vi "Launcher (Top Level).vi"(8 "Error In":errorcluster) -> (0 "Error Out":errorcluster)   [LabVIEW 2015]
doc: "This VI is used to launch all modules to run in parallel. Each module has APIs to do its own operation \nand send and receive data from other modules."
uses:
  User Events/Controls/User Events States.ctl
  Modules/Config Database/Config DB.lvlib
  Modules/Vehicle Position Interface/Vehicle Position Interface.lvlib
  Modules/Wash Display Console/Wash Display Console.lvlib
  Modules/Entry Console/Entry Console.lvlib
  Modules/Controller/Controller.lvlib
  Modules/Error Handler/Error Handler.lvlib
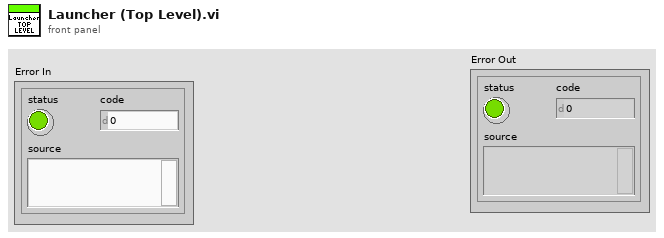
[diagram p1: front panel]
types:
  T1 = typedef "User Events States.ctl" = enum16{"Get", "Create", "Destroy"}
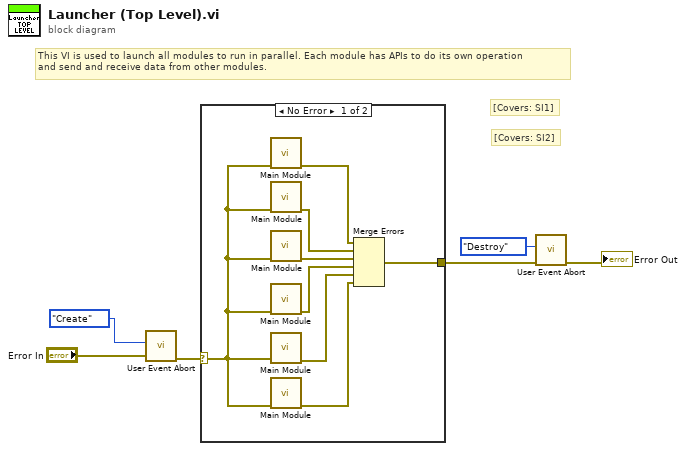
[diagram p0: block diagram]
diagram:
  # "[Covers: SI2]"
  # "[Covers: SI1]"
  # "This VI is used to launch all modules to run in parallel. Each module has APIs to do its own operation \nand send and receive data from other modules."
  n1 = call "User Event Abort.vi"("Error In"="Error In", "User Event States"=User_Events_States."Create") -> ("Error Out"=w4:errorcluster)  [unwired: 8 in, 1 out]
  n2 = case shown="No Error" w4 {
    selector: w4 -> [w8 w15]
    tunnel: [w9 w15] -> w1
    frame No Error {
      n3 = call "Main Module.vi"("Error In"=w8) -> ("Error Out"=w14:errorcluster)  [unwired: 10 in]
      n4 = call "Main Module.vi"("Error In"=w8) -> ("Error Out"=w13:errorcluster)  [unwired: 10 in]
      n5 = call "Main Module.vi"("Error In"=w8) -> ("Error Out"=w12:errorcluster)  [unwired: 10 in]
      n6 = call "Main Module.vi"("Error In"=w8) -> ("Error Out"=w11:errorcluster)  [unwired: 10 in]
      n7 = call "Main Module.vi"("Error In"=w8) -> ("Error Out"=w10:errorcluster)  [unwired: 10 in]
      n8 = call "Main Module.vi"("Error In"=w8) -> ("Error Out"=w7:errorcluster)  [unwired: 10 in]
      n9 = Merge Errors(w14, w13, w12, w11, w10, w7) -> (w9:errorcluster)
    }
    frame Error {
    }
  }
  n10 = call "User Event Abort.vi"("Error In"=w1, "User Event States"=User_Events_States."Destroy") -> ("Error Out"=→"Error Out":errorcluster)  [unwired: 8 in, 1 out]
